vi "Timestamp.vi"() -> (2 "Date/time String":string)   [LabVIEW 2018, in "TracerLibrary.lvlib" / "Tracer.lvclass"]
uses:
  Tracer.lvclass
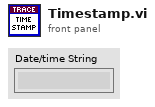
[diagram p1: front panel]
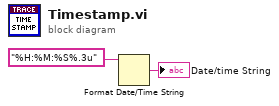
[diagram p0: block diagram]
diagram:
  n1 = Format Date/Time String(time format string (%c)="%H:%M:%S%.3u") -> (date/time string=→"Date/time String":string)  [unwired: 2 in]
